vi "fgv_agv_config.vi"(7 "cmd":enum16{"read", "write"}(ring), 8 "error in":errorcluster, 11 "AGV cfg":T1={"Port"="COM6", "speed limits"={"speed-limit"=0.1, "steer-limit"=0.0}, "limits"={"speed limits"={"max"=0.1, "min"=0.0}, "steer limits"={"max"=0.1, "min"=0.0}}}) -> (0 "error out":errorcluster, 3 "AGV cfg out":T1={"Port"="COM6", "speed limits"={"speed-limit"=0.1, "steer-limit"=0.0}, "limits"={"speed limits"={"max"=0.1, "min"=0.0}, "steer limits"={"max"=0.1, "min"=0.0}}})   [LabVIEW 2019]
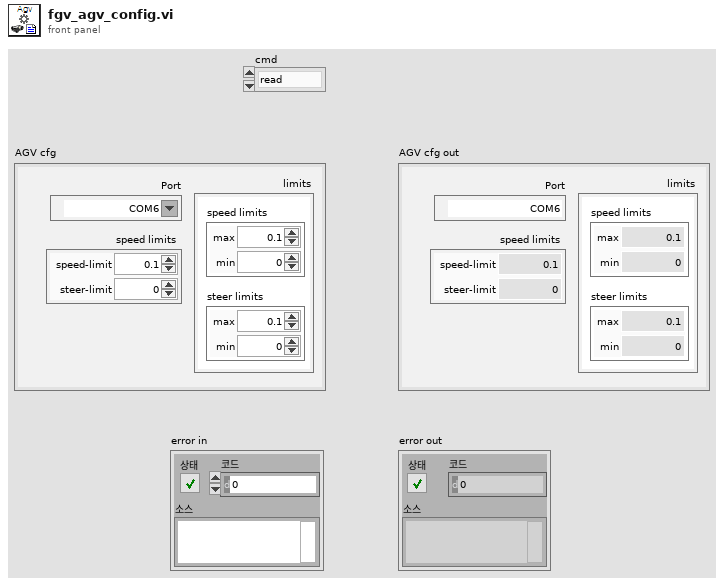
[diagram p1: front panel]
types:
  T1 = cluster{"Port":refnum<visa-resource-name>, "speed limits":cluster{"speed-limit":dbl, "steer-limit":dbl}, "limits":cluster{"speed limits":cluster{"max":dbl, "min":dbl}, "steer limits":cluster{"max":dbl, "min":dbl}}}
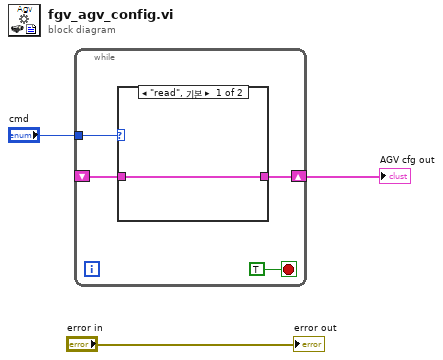
[diagram p0: block diagram]
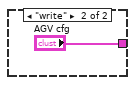
[diagram p2: hidden frame]
diagram:
  n1 = while {
    tunnel: "cmd" -> [w6]
    shift-right: [w5] -> w1
    shift-left: _ -> [w4]
    stop <- TRUE stop-if-true
    n2 = case shown="\"read\", 기본" w6 {
      tunnel: [w8 "AGV cfg"] -> w5
      tunnel: w4 -> [w8 _]
      frame "read", Default {
      }
      frame "write" {
      }
    }
  }
  "AGV cfg out" <- w1
  "error out" <- "error in"
